vi "Server_Create Listener.vi"(8 "error in":errorcluster) -> (0 "error out":errorcluster)   [LabVIEW 2018, in "Cloud Server.lvlib"]
uses:
  Cloud Server.lvlib
  Data Def/Server_FGV Method.ctl
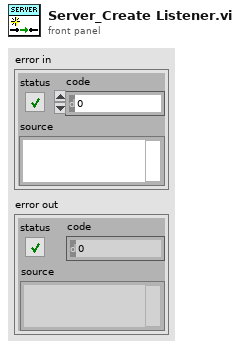
[diagram p1: front panel]
types:
  T1 = typedef "Cloud Server.lvlib/Server_FGV Method.ctl" = enum16{"Get", "Put"}
  T2 = typedef "Cloud Server.lvlib/Server_Main Data.ctl" = cluster{"Main VI Ref.":refnum<vi>, "Listener ID":refnum<k5>, "Meta data":T3[], "Main Queue":T5, "User Picture":T6}
  T3 = typedef "stm_MetaElement.ctl" = cluster{"Name":T4}
  T4 = typedef "stm_MetaDataElement.ctl" = string
  T5 = typedef "Cloud Server.lvlib/Server_Main Queue.ctl" = cluster{"Server Write Queue":refnum<queue>, "Main Loop Queue":refnum<queue>}
  T6 = typedef "IMAQ Image.ctl" = refnum<image>
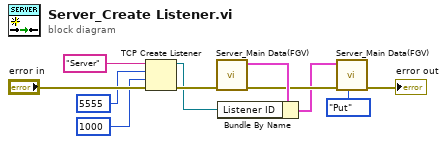
[diagram p0: block diagram]
diagram:
  n1 = TCP Create Listener(8:"error in", 9:1000 ("timeout ms (25000)"), 10:u16 5555 ("port"), 11:"Server" ("service name")) -> (0:w7:errorcluster, 3:w5:refnum<k5>)  [unwired: 1 in, 1 out]
  n2 = call "Server_Main Data(FGV).vi"("error in"=w7) -> ("error out"=w4:errorcluster, "Main Data Out"=w6:T2)  [unwired: 9 in]
  n3 = Bundle By Name(cluster=w6, "Listener ID"=w5) -> (w3:T2)
  n4 = call "Server_Main Data(FGV).vi"("FGV Method(Get)"=Server_FGV_Method."Put", "error in"=w4, "Main Data In"=w3) -> ("error out"=→"error out":errorcluster)  [unwired: 7 in, 1 out]
